vi "DG535.get outputs settings.vi"(0 "i ref in":refnum<vi>, 5 "read":bool, 7 "output":i32(ring) items=["T0", "A", "B", "AB", "C", "D", "CD"], 11 "error in (no error)":errorcluster) -> (3 "mode":i32(ring) items=["TTL", "NIM", "ECL", "VAR"], 4 "i ref out":refnum<vi>, 6 "amplitude":dbl=1.0 min=-3.0 max=4.0 format="%.2f", 8 "offset":dbl min=-3.0 max=4.0 format="%.2f", 10 "load":bool, 14 "inversion":bool, 15 "error out":errorcluster)   [LabVIEW 2014, in "DG535.lvlib"]
doc: "This vi is used ti retrieve the Mode, AMplitude, Offset, Load and Inversion parameters of a selected ouputs while pressing \"read\"."
uses:
  DG535.lvlib
panel:
  # "50 Ohms"
  # "High Z"
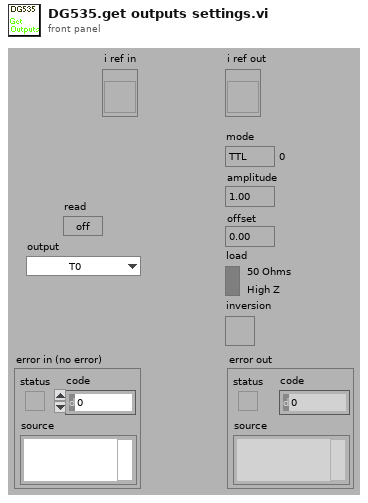
[diagram p1: front panel]
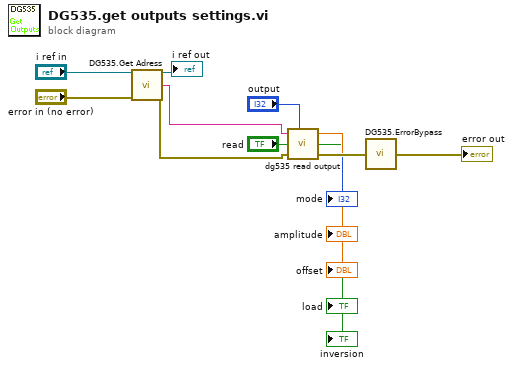
[diagram p0: block diagram]
diagram:
  n1 = call "DG535.Get Adress.vi"("i ref in"="i ref in", "error in (no error)"="error in (no error)") -> ("i ref out"=→"i ref out":refnum<vi>, "address"=w9:string, "error out"=w8:errorcluster)  [unwired: 10 in, 1 out]
  n2 = call "dg535 read output.vi"("GPIB address"=w9, "output"="output", "read"="read", "error in"=w8) -> ("mode"=→"mode":i32, "offset"=→"offset":dbl, "amplitude"=→"amplitude":dbl, "inversion"=→"inversion":bool, "load"=→"load":bool, "error out"=w7:errorcluster)
  n3 = call "DG535.ErrorBypass.vi"("error in (no error)"=w7) -> ("error out"=→"error out":errorcluster)  [unwired: 14 in]
